vi "WSVCAP SHL FPGA LL SPI Write Data.vi"(0 "Bit In":bool, 7 "Data Word In":u16, 11 "error in (no error)":errorcluster, 12 "Socket Mask":u16, 13 "Line":T1) -> (15 "error out":errorcluster)   [LabVIEW 2012]
uses:
  Type Defs/WSVCAP SHL SPI Write Line Enum.ctl
  <vilib>/rvi/eio/common/nirviEmuTemplateMethod_errors.vi
  <vilib>/eio/EIONode/EIONode.xnode
  WSVCAP SHL FPGA LL SPI Debug Global.vi
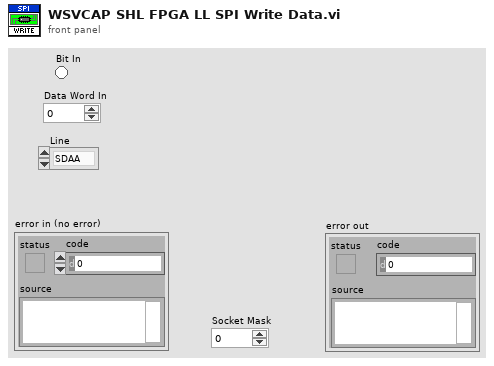
[diagram p1: front panel]
types:
  T1 = typedef "WSVCAP SHL SPI Write Line Enum.ctl" = enum16{"SDAA", "SDEN", "SCLK"}
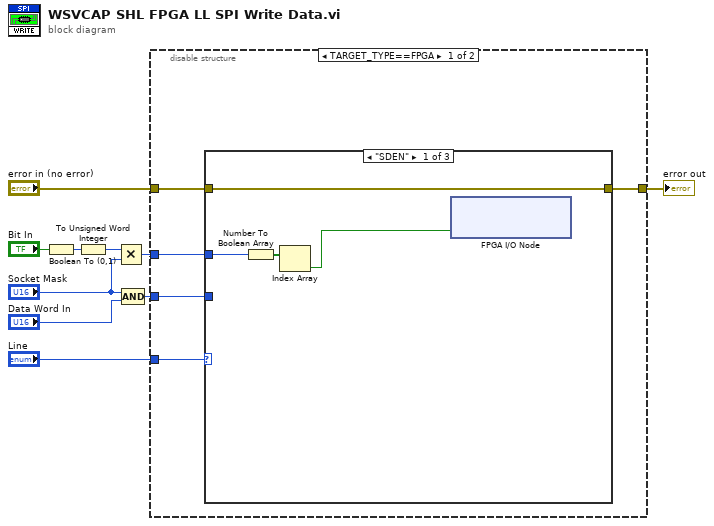
[diagram p0: block diagram]
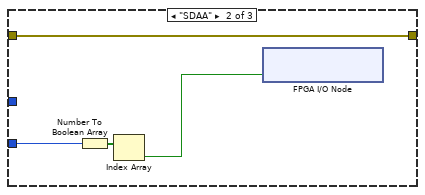
[diagram p2: hidden frame]
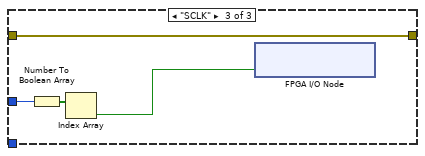
[diagram p3: hidden frame]
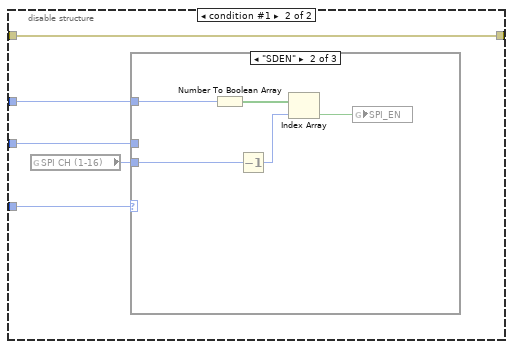
[diagram p4: hidden frame]
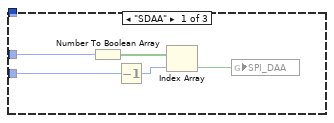
[diagram p5: hidden frame]
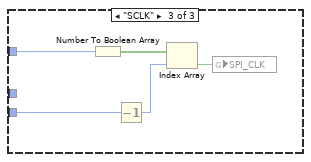
[diagram p6: hidden frame]
diagram:
  n1 = Boolean To (0,1)(Boolean="Bit In") -> (0, 1=w4:i16)
  n2 = To Unsigned Word Integer(number=w4) -> (unsigned 16bit integer=w3:u16)
  n3 = Multiply(x=w3, y="Socket Mask") -> (x*y=w1:u16)
  n4 = Compound Arithmetic op=AND("Socket Mask", "Data Word In") -> (w6:u16)
  n5 = disable-structure shown="TARGET_TYPE==FPGA" {
    disable-tunnel: "Line" -> [w15 w32]
    disable-tunnel: [w14 w31] -> w9
    disable-tunnel: "error in (no error)" -> [w13 w31]
    disable-tunnel: w6 -> [w12 w30]
    disable-tunnel: w1 -> [w11 w28]
    frame condition #0 (active) {
      n6 = case shown="\"SDEN\"" w15 {
        tunnel: [w16 w21 w24] -> w14
        tunnel: w13 -> [w16 w21 w24]
        tunnel: w12 -> [_ w23 _]
        tunnel: w11 -> [w18 _ w26]
        frame "SDEN" {
          n7 = Number To Boolean Array(number=w18) -> (Boolean array=w19:bool[])
          n8 = Index Array(array=w19) -> (element=w17:bool)  [unwired: 1 in]
          n9 = xnode "FPGA I/O Node"("I2C_SDA_C1_S1"=w17) -> ()  [unwired: 2 in, 2 out]
        }
        frame "SDAA" {
          n10 = Number To Boolean Array(number=w23) -> (Boolean array=w22:bool[])
          n11 = Index Array(array=w22) -> (element=w20:bool)  [unwired: 1 in]
          n12 = xnode "FPGA I/O Node"("I2C_SDA_C1_S1"=w20) -> ()  [unwired: 1 in, 1 out]
        }
        frame "SCLK" {
          n13 = Number To Boolean Array(number=w26) -> (Boolean array=w27:bool[])
          n14 = Index Array(array=w27) -> (element=w25:bool)  [unwired: 1 in]
          n15 = xnode "FPGA I/O Node"("I2C_SDA_C1_S1"=w25) -> ()  [unwired: 1 in, 1 out]
        }
      }
    }
    frame condition #1 {
      n16 = global read "WSVCAP SHL FPGA LL SPI Debug Global.vi" "SPI CH (1-16)"() -> (w29:i32)
      n17 = case shown="\"SDEN\"" w32 {
        tunnel: w30 -> [w34 _ _]
        tunnel: w29 -> [w33 w40 w45]
        tunnel: w28 -> [_ w38 w43]
        frame "SDAA" {
          n18 = Number To Boolean Array(number=w34) -> (Boolean array=w37:bool[])
          n19 = Decrement(x=w33) -> (x-1=w35:i32)
          n20 = Index Array(array=w37, index=w35) -> (element=w36:bool)
          n21 = global write "WSVCAP SHL FPGA LL SPI Debug Global.vi" "SPI_DAA"(w36) -> ()
        }
        frame "SDEN" {
          n22 = Number To Boolean Array(number=w38) -> (Boolean array=w42:bool[])
          n23 = Decrement(x=w40) -> (x-1=w41:i32)
          n24 = Index Array(array=w42, index=w41) -> (element=w39:bool)
          n25 = global write "WSVCAP SHL FPGA LL SPI Debug Global.vi" "SPI_EN"(w39) -> ()
        }
        frame "SCLK" {
          n26 = Number To Boolean Array(number=w43) -> (Boolean array=w47:bool[])
          n27 = Decrement(x=w45) -> (x-1=w46:i32)
          n28 = Index Array(array=w47, index=w46) -> (element=w44:bool)
          n29 = global write "WSVCAP SHL FPGA LL SPI Debug Global.vi" "SPI_CLK"(w44) -> ()
        }
      }
    }
  }
  "error out" <- w9
